vi "SingleJointedArmSim_example.vi"() -> ()   [LabVIEW 2019]
uses:
  <vilib>/Rock Robotics/WPI/ThirdParty/JAS_Junk/TrajLib/DCMOTOR.CTL
  <vilib>/Rock Robotics/WPI/ThirdParty/JAS_Junk/TrajLib/LINEAR_SYSTEM.ctl
  <vilib>/Analysis/Matrix/Datatypes/RealMatrix.ctl
  <vilib>/Rock Robotics/WPI/ThirdParty/JAS_Junk/TrajLib/LINEAR_QUADRATIC_REGULATOR.ctl
  <vilib>/Rock Robotics/WPI/ThirdParty/JAS_Junk/TrajLib/KALMAN_FILTER.ctl
  <vilib>/Rock Robotics/WPI/ThirdParty/JAS_Junk/TrajLib/LINEAR_SYSTEM_LOOP.ctl
  <vilib>/Rock Robotics/WPI/ThirdParty/JAS_Junk/TrajLib/LINEAR_PLANT_INV_FF.ctl
  <vilib>/Rock Robotics/WPI/ThirdParty/JAS_Junk/TrajLib/SINGLE_JOINT_ARM_SIM.ctl
  <vilib>/Rock Robotics/WPI/ThirdParty/JAS_Junk/TrajLib/LINEAR_SYSTEM_SIM.ctl
  <vilib>/numeric/Random Number (Range) DBL.vi
  <vilib>/Rock Robotics/WPI/ThirdParty/JAS_Junk/TrajLib/MatBuilder_Create.vi
  <vilib>/Rock Robotics/WPI/ThirdParty/JAS_Junk/TrajLib/DCMotor_New.vi
  <vilib>/Rock Robotics/WPI/ThirdParty/JAS_Junk/TrajLib/Units_RotationsPerMinuteToRadiansPerSecond.vi
  <vilib>/Rock Robotics/WPI/ThirdParty/JAS_Junk/TrajLib/LinearSystem_New.vi
  <vilib>/Rock Robotics/WPI/ThirdParty/JAS_Junk/TrajLib/MatrixHelper_Zero.vi
  <vilib>/Rock Robotics/WPI/ThirdParty/JAS_Junk/TrajLib/MatBuilder_Fill.vi
  <vilib>/Rock Robotics/WPI/ThirdParty/JAS_Junk/TrajLib/MatrixHelper_CoerceSize.vi
  <vilib>/Rock Robotics/WPI/ThirdParty/JAS_Junk/TrajLib/Trajectory_Library.lvlib
  <vilib>/Analysis/Matrix/NI_Matrix.lvlib
panel:
  in  "Tab Control":T1(tab)
  out "Arm Motor":T2 {"Kt_NMPerAmp" format="%13.5p"; "Kv_RadPerSecPerVolt" format="%13.5p"; "R_Ohms" format="%13.5p"; "FreeSpeed_RadPerSec" format="%13.5p"; "FreeCurrent_Amps" format="%13.5p"; "StallCurrent_Amps" format="%13.5p"; "StallTorque_NM" format="%13.5p"; "nominalVoltage_Volts" format="%13.5p"}
  out "m_Arm":T3
  out "KalmanFilter":T5
  out "Kalman Error":bool
  out "LinearQuadraticRegulator":T6
  out "LQR Error":bool
  out "Linear System Loop":T7
  out "LinSysLoop_Error":bool
  out "Single Joint Arm Simulaation":T9 {"GearBox"."Kt_NMPerAmp" format="%13.5p"; "GearBox"."Kv_RadPerSecPerVolt" format="%13.5p"; "GearBox"."R_Ohms" format="%13.5p"; "GearBox"."FreeSpeed_RadPerSec" format="%13.5p"; "GearBox"."FreeCurrent_Amps" format="%13.5p"; "GearBox"."StallCurrent_Amps" format="%13.5p"; "GearBox"."StallTorque_NM" format="%13.5p"; "GearBox"."nominalVoltage_Volts" format="%13.5p"}
  out "Shooting A":T4
  out "Shooting B":T4
  out "Battery Voltage":dbl format="%20.3f"
  in  "Extra weight":bool
  out "CO Chart":cluster{dbl, "Voltage":dbl}(graph)
  in  "GO UP":bool
  out "Encoer Speed\nRad/Sec":dbl(slide) scale=-1.0..6.0
  out "Height":dbl format="%20.3f"
  out "Cor Err":bool
  out "Kalman Filtered\nHeight":dbl format="%20.3f"
  out "PV Chart":T11(graph)
  out "Predict Err":bool
  out "Motor Volt Dmd (CO)":dbl format="%20.3f"
  out "At Top":bool
  out "At Bottom":bool
  out "Motor Amps":dbl format="%20.3f"
  # "<States,States>"
  # "<States,Inputs>"
  # "<Outputs,States>"
  # "<Outputs,Inputs>"
  # "Steady State Gain  \n<States,Outputs>"
  # "State Estimate <Statess,1>"
  # "<States,States>"
  # "<States,Inputs>"
  # "<Outputs,States>"
  # "<Outputs,Inputs>"
  # "Ref State <States,1>"
  # "Comp and capped \noutput <Inputs,1>"
  # "Controller gain\n<Inputs,States>"
  # "<States,1>"
  # "<FUTURE --- CLAMP TYPE -- For now\nuse Normalize>"
  # "Steady State Gain  \n<States,Outputs>"
  # "State Estimate <Statess,1>"
  # "<States,States>"
  # "<States,Inputs>"
  # "<Outputs,States>"
  # "<Outputs,Inputs>"
  # "<States,1>"
  # "<Inputs,1>"
  # "<States,Inputs>"
  # "<States,States>"
  # "Ref State <States,1>"
  # "Comp and capped \noutput <Inputs,1>"
  # "Controller gain\n<Inputs,States>"
  # "<States, 1>"
  # "<Outputs, 1>"
  # "<Inputs, 1>"
  # "<Outputs, 1>"
  # "<States,States>"
  # "<States,Inputs>"
  # "<Outputs,States>"
  # "<Outputs,Inputs>"
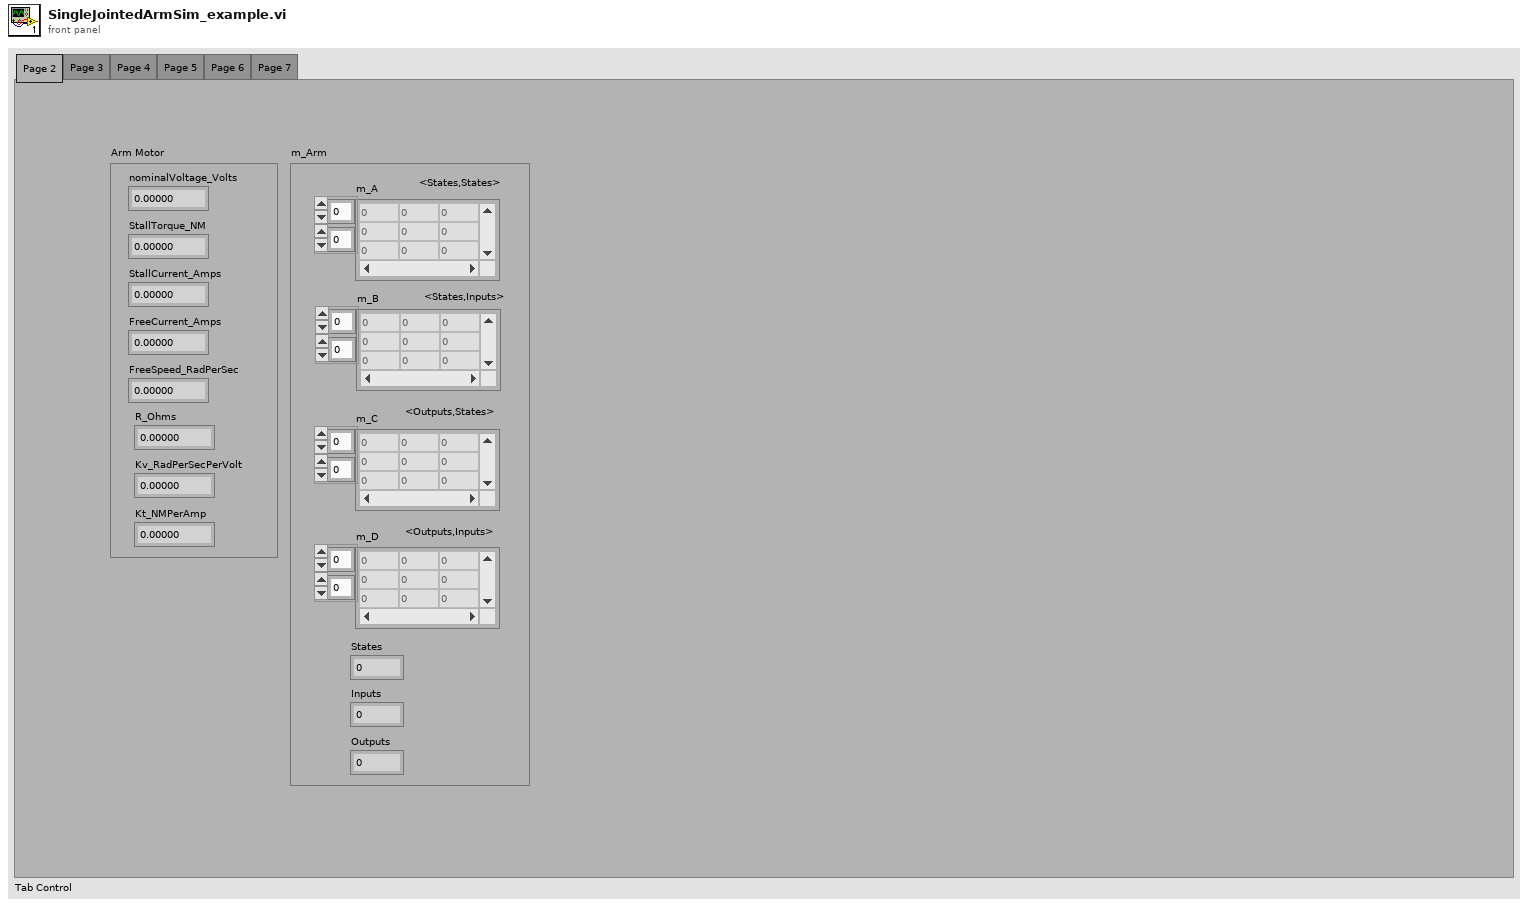
[diagram p1: front panel]
types:
  T1 = enum32{"Page 2", "Page 3", "Page 4", "Page 5", "Page 6", "Page 7"}
  T2 = typedef "Trajectory_Library.lvlib/DCMOTOR.CTL" = cluster{"nominalVoltage_Volts":dbl, "StallTorque_NM":dbl, "StallCurrent_Amps":dbl, "FreeCurrent_Amps":dbl, "FreeSpeed_RadPerSec":dbl, "R_Ohms":dbl, "Kv_RadPerSecPerVolt":dbl, "Kt_NMPerAmp":dbl}
  T3 = typedef "Trajectory_Library.lvlib/LINEAR_SYSTEM.ctl" = cluster{"m_A":T4, "m_B":T4, "m_C":T4, "m_D":T4, "States":i32, "Inputs":i32, "Outputs":i32}
  T4 = typedef "NI_Matrix.lvlib/RealMatrix.ctl" = dbl[][]
  T5 = typedef "Trajectory_Library.lvlib/KALMAN_FILTER.ctl" = cluster{"m_K":T4, "m_xHat":T4, "States":i32, "Outputs":i32, "m_Plant":T3}
  T6 = typedef "Trajectory_Library.lvlib/LINEAR_QUADRATIC_REGULATOR.ctl" = cluster{"m_r":T4, "m_U":T4, "m_K":T4, "States":i32, "Inputs":i32}
  T7 = typedef "Trajectory_Library.lvlib/LINEAR_SYSTEM_LOOP.ctl" = cluster{"Controller":T6, "FeedForward":T8, "Observer":T5, "Next_R":T4, "Clamp Max":T4}
  T8 = typedef "Trajectory_Library.lvlib/LINEAR_PLANT_INV_FF.ctl" = cluster{"m_R":T4, "m_Uff":T4, "m_B":T4, "m_A":T4, "States":i32, "Inputs":i32}
  T9 = typedef "Trajectory_Library.lvlib/SINGLE_JOINT_ARM_SIM.ctl" = cluster{"Arm_LinearSystem":T10, "GearBox":T2, "Gearing":dbl, "R_ArmLength_M":dbl, "MinAngle_M":dbl, "MaxAngle_M":dbl, "ArmMass_Kg":dbl, "SimulateGravity":bool}
  T10 = typedef "Trajectory_Library.lvlib/LINEAR_SYSTEM_SIM.ctl" = cluster{"m_Plant":T3, "m_X":T4, "m_Y":T4, "m_U":T4, "MeasureStdDev":T4}
  T11 = cluster{"upper limit":dbl, "Real Matrix Element":dbl, "Real Matrix Element":dbl}
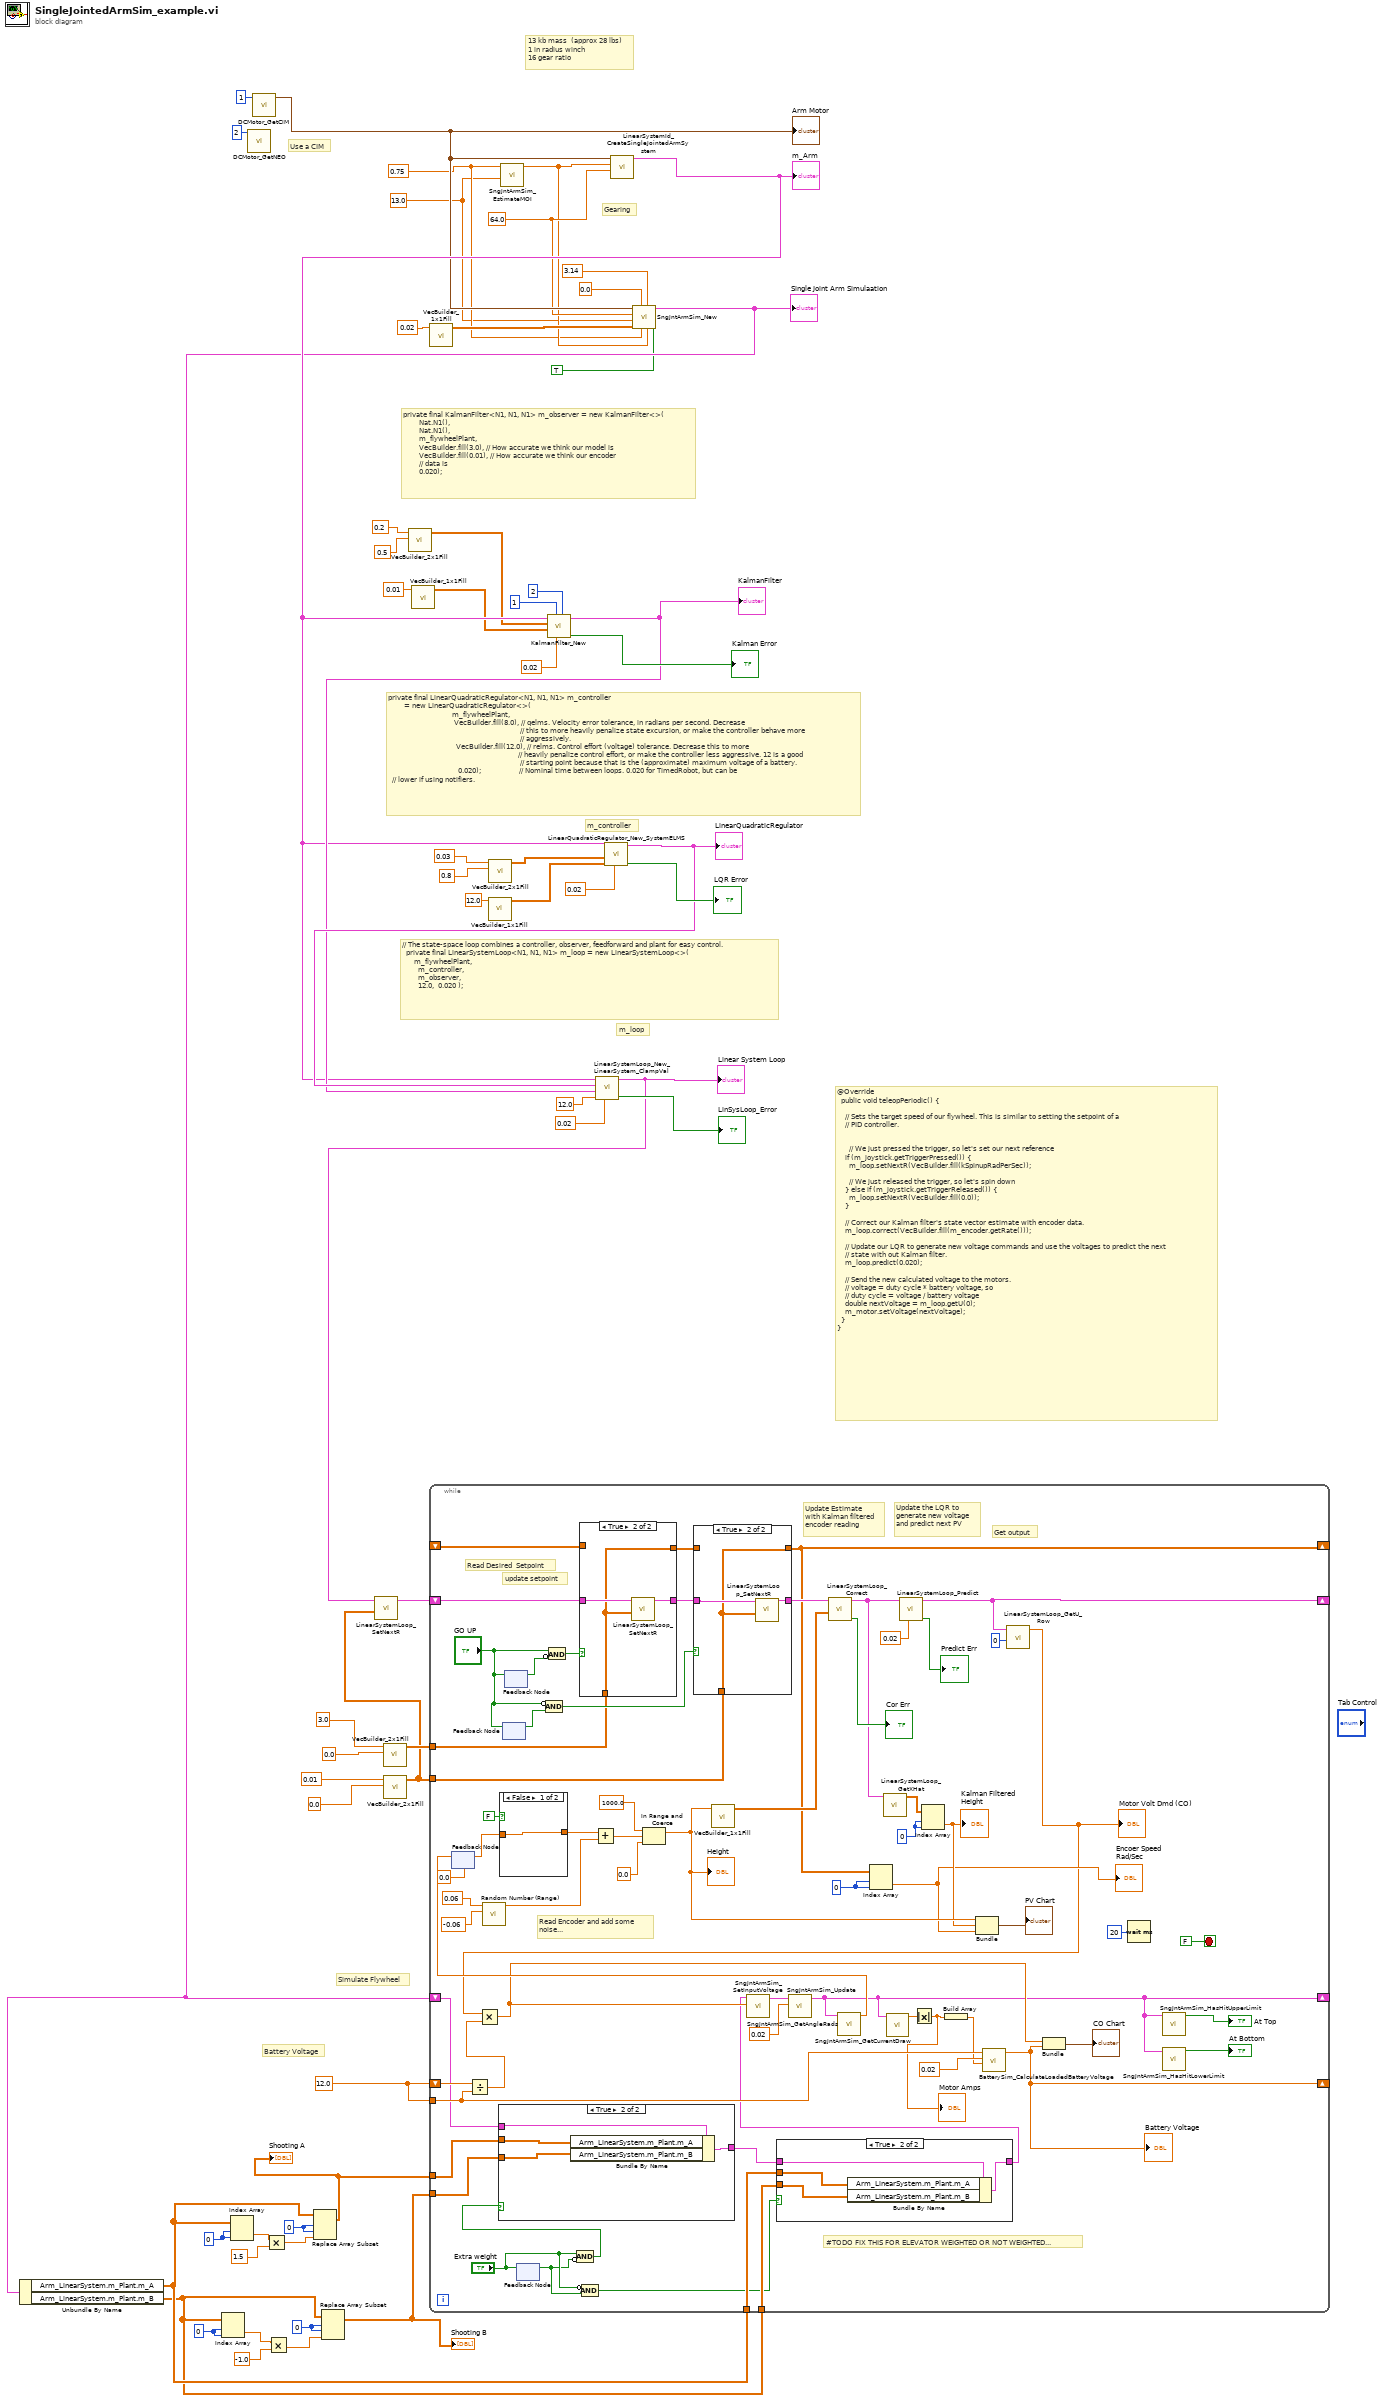
[diagram p0: block diagram]
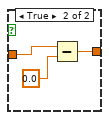
[diagram p4: hidden frame]
diagram:
  w3 = 0.75 ("ArmLength_M")
  w23 = 0 ("index (row)")
  w24 = 0 ("index (row)")
  w25 = 0 ("index (row)")
  w26 = 0 ("index (row)")
  w6 = 64.0 ("G")
  w2 = 13.0 ("massKg")
  w50 = 12.0
  # "Simulate Flywheel"
  # "m_loop"
  # "m_controller"
  # "13 kb mass  (approx 28 lbs)\n1 in radius winch\n16 gear ratio"
  # "Gearing"
  # "Use a CIM"
  # "Battery Voltage"
  # "@Override\n  public void teleopPeriodic() {\n\n    // Sets the target speed of our flywheel. This is similar to setting the setpoint of a\n    // PID controller.\n\n\n      // We just pressed the trigger, so let's set our next reference\n    if (m_joystick.getTriggerPressed()) {\n      m_loop.setNextR(VecBuilder.fill(kSpinupRadPerSec));\n\n      // We just released the trigger, so let's spin down\n    } else if (m_joystick.getTriggerReleased()) {\n      m_loop.setNextR(VecBuilder.fill(0.0));\n    }\n\n    // Correct our Kalman filter's state vector estimate with encoder data.\n    m_loop.correct(VecBuilder.fill(m_encoder.getRate()));\n\n    // Update our LQR to generate new voltage commands and use the voltages to predict the next\n    // state with out Kalman filter.\n    m_loop.predict(0.020);\n\n    // Send the new calculated voltage to the motors.\n    // voltage = duty cycle * battery voltage, so\n    // duty cycle = voltage / battery voltage\n    double nextVoltage = m_loop.getU(0);\n    m_motor.setVoltage(nextVoltage);\n  }\n}"
  # "// The state-space loop combines a controller, observer, feedforward and plant for easy control.\n  private final LinearSystemLoop<N1, N1, N1> m_loop = new LinearSystemLoop<>(\n      m_flywheelPlant,\n        m_controller,\n        m_observer,\n        12.0,  0.020 );"
  # "private final LinearQuadraticRegulator<N1, N1, N1> m_controller\n        = new LinearQuadraticRegulator<>(\n                                m_flywheelPlant,\n                                 VecBuilder.fill(8.0), // qelms. Velocity error tolerance, in radians per second. Decrease\n                                                                  // this to more heavily penalize state excursion, or make the controller behave more\n                                                                  // aggressively.\n                                  VecBuilder.fill(12.0), // relms. Control effort (voltage) tolerance. Decrease this to more\n                                                                 // heavily penalize control effort, or make the controller less aggressive. 12 is a good\n                                                                  // starting point because that is the (approximate) maximum voltage of a battery.\n                                   0.020);                   // Nominal time between loops. 0.020 for TimedRobot, but can be\n  // lower if using notifiers."
  # "private final KalmanFilter<N1, N1, N1> m_observer = new KalmanFilter<>(\n        Nat.N1(), \n        Nat.N1(),\n        m_flywheelPlant,\n        VecBuilder.fill(3.0), // How accurate we think our model is\n        VecBuilder.fill(0.01), // How accurate we think our encoder\n        // data is\n        0.020);"
  n1 = call <vilib>:"DCMotor_GetNEO.vi"("Num Motors"=2) -> ()  [unwired: 10 in, 1 out]
  n2 = call <vilib>:"DCMotor_GetCIM.vi"("Num Motors"=1) -> ("DCMOTOR"=w9:T2)  [unwired: 10 in]
  "Arm Motor" <- w9
  n3 = call <vilib>:"VecBuilder_2x1Fill.vi"("R1"=0.0, "R0"=3.0 ("RotationsPerMinute")) -> ("output matrix"=w16:T4)  [unwired: 9 in]
  n4 = call <vilib>:"VecBuilder_2x1Fill.vi"("R1"=0.0, "R0"=0.01 ("R0_C0")) -> ("output matrix"=w11:T4)  [unwired: 9 in]
  n5 = call <vilib>:"VecBuilder_2x1Fill.vi"("R1"=0.5, "R0"=0.2 ("R0_C0")) -> ("output matrix"=w37:T4)  [unwired: 9 in]
  n6 = call <vilib>:"VecBuilder_1x1Fill.vi"("R0_C0"=0.01) -> ("output matrix"=w36:T4)  [unwired: 10 in]
  n7 = call <vilib>:"VecBuilder_1x1Fill.vi"("R0_C0"=0.02) -> ("output matrix"=w5:T4)  [unwired: 10 in]
  n8 = call <vilib>:"VecBuilder_1x1Fill.vi"("R0_C0"=12.0) -> ("output matrix"=w30:T4)  [unwired: 10 in]
  n9 = call <vilib>:"VecBuilder_2x1Fill.vi"("R1"=0.8 ("R0_C0"), "R0"=0.03 ("R0_C0")) -> ("output matrix"=w32:T4)  [unwired: 9 in]
  n10 = call <vilib>:"SngJntArmSim_EstimateMOI.vi"("ArmMass_Kg"=w2, "ArmLength_M"=w3) -> ("MOI"=w4:dbl)  [unwired: 9 in]
  n11 = call <vilib>:"LinearSystemId_CreateSingleJointedArmSystem.vi"("G"=w6, "jKgSquaredMeters"=w4, "DCMOTOR"=w9) -> ("Linearsystem"=w44:T3)  [unwired: 8 in]
  "m_Arm" <- w44
  n12 = call <vilib>:"KalmanFilter_New.vi"("States"=2, "dt_Seconds"=0.02, "Outputs"=1, "MeasurementStdDevs"=w36, "StateStdDevs"=w37, "Plant"=w44) -> ("Error"=→"Kalman Error":bool, "KalmanFilter"=w54:T5)  [unwired: 4 in]
  "KalmanFilter" <- w54
  n13 = call <vilib>:"LinearQuadraticRegulator_New_SystemELMS.vi"("dt_Seconds"=0.02, "Relms"=w30, "Qelms"=w32, "LINEARSYSTEM"=w44) -> ("Error"=→"LQR Error":bool, "LinearQuadraticRegulator"=w55:T6)  [unwired: 6 in]
  "LinearQuadraticRegulator" <- w55
  n14 = call <vilib>:"LinearSystemLoop_New_LinearSystem_ClampVal.vi"("dT_Seconds"=0.02, "Max_Voltage"=12.0, "Observer"=w54, "Controller"=w55, "Plant"=w44) -> ("Error"=→"LinSysLoop_Error":bool, "Linear System Loop"=w12:T7)  [unwired: 5 in]
  "Linear System Loop" <- w12
  n15 = call <vilib>:"LinearSystemLoop_SetNextR.vi"("R"=w11, "input inear System Loop"=w12) -> ("out Linear System Loop"=w13:T7)  [unwired: 9 in]
  n16 = call <vilib>:"SngJntArmSim_New.vi"("SimulateGravity"=TRUE, "jKgMetersSquared"=w4, "MaxAngle_Rad"=3.14 ("MaxHeight_Meters"), "ArmLength_Meters"=w3, "MinAngle_Rad"=0.0 ("MinHeight_Meters"), "MeasurementStdDev"=w5, "ArmMass_Kg"=w2, "Gearing"=w6, "GearBox"=w9) -> ("SingleJointArmSim"=w10:T9)  [unwired: 2 in]
  "Single Joint Arm Simulaation" <- w10
  n17 = Unbundle By Name(w10) -> ("Arm_LinearSystem.m_Plant.m_A"=w48:T4, "Arm_LinearSystem.m_Plant.m_B"=w47:T4)
  n18 = Index Array(array=w47, index (row)=w26, index (col)=w26) -> (element=w18:dbl)
  n19 = Index Array(array=w48, index (row)=w25, index (col)=w25) -> (element=w22:dbl)
  n20 = Multiply(x=w22, y=1.5) -> (x*y=w20:dbl)
  n21 = Multiply(x=w18, y=-1.0) -> (x*y=w17:dbl)
  n22 = Replace Array Subset(array=w48, new element=w20, index (row)=w23, index (col)=w23) -> (w46:T4)
  "Shooting A" <- w46
  n23 = Replace Array Subset(array=w47, new element=w17, index (row)=w24, index (col)=w24) -> (w45:T4)
  "Shooting B" <- w45
  n24 = while {
    shift-right: [w68] -> _
    shift-left: w13 -> [w118]
    tunnel: w16 -> [w116]
    tunnel: w11 -> [w115]
    shift-right: [w59] -> _
    shift-left: w10 -> [w76]
    shift-right: [w90] -> _
    shift-left: _ -> [w91]
    shift-right: [w78] -> _
    shift-left: w50 -> [w85]
    tunnel: w50 -> [w82]
    tunnel: w48 -> [w72]
    tunnel: w47 -> [w71]
    tunnel: w46 -> [w70]
    tunnel: w45 -> [w69]
    stop <- FALSE stop-if-true
    w89 = 0 ("index (row)")
    w105 = 0 ("index (row)")
    # "#TODO FIX THIS FOR ELEVATOR WEIGHTED OR NOT WEIGHTED..."
    # "Get output"
    # "Update the LQR to \ngenerate new voltage\nand predict next PV"
    # "update setpoint"
    # "Read Desired  Setpoint"
    # "Update Estimate\nwith Kalman filtered\nencoder reading"
    # "Read Encoder and add some \nnoise..."
    n25 = feedback #1(0.0 ("Velocity_RadPerSec")) -> (w87:dbl)
    n26 = Divide(x=w85, y=w82) -> (x/y=w83:dbl)
    n27 = call-poly <vilib>:"Random Number (Range).vi"("lower bound (0)"=-0.06, "upper bound (100)"=0.06) -> ("number"=w112:dbl)  [unwired: 9 in]
    n28 = case shown="False" FALSE {
      tunnel: w87 -> [w136 w139]
      tunnel: [w136 w138] -> w86
      frame False {
      }
      frame True {
        n29 = Subtract(x=w139, y=0.0) -> (x-y=w138:dbl)
      }
    }
    n30 = feedback #2() -> (w122:bool)  [unwired: 1 in]
    n31 = feedback-in #2("GO UP") -> ()
    n32 = feedback-in #3("GO UP") -> ()
    n33 = feedback #3() -> (w123:bool)  [unwired: 1 in]
    n34 = feedback-in #4("Extra weight") -> ()
    n35 = feedback #4() -> (w64:bool)  [unwired: 1 in]
    n36 = Compound Arithmetic op=AND(invert "GO UP", w122) -> (w119:bool)
    n37 = Compound Arithmetic op=AND("GO UP", invert w123) -> (w120:bool)
    n38 = Compound Arithmetic op=AND("Extra weight", invert w64) -> (w73:bool)
    n39 = case shown="True" w73 {
      tunnel: w76 -> [w131 w135]
      tunnel: [w131 w132] -> w75
      tunnel: w70 -> [_ w134]
      tunnel: w69 -> [_ w133]
      frame False {
      }
      frame True {
        n40 = Bundle By Name(cluster=w135, "Arm_LinearSystem.m_Plant.m_A"=w134, "Arm_LinearSystem.m_Plant.m_B"=w133) -> (w132:T9)
      }
    }
    n41 = case shown="True" w120 {
      tunnel: w118 -> [w146 w148]
      tunnel: [w146 w149] -> w117
      tunnel: w116 -> [_ w147]
      tunnel: [w145 w147] -> w92
      tunnel: w91 -> [w145 _]
      frame False {
      }
      frame True {
        n42 = call <vilib>:"LinearSystemLoop_SetNextR.vi"("R"=w147, "input inear System Loop"=w148) -> ("out Linear System Loop"=w149:T7)  [unwired: 9 in]
      }
    }
    n43 = Compound Arithmetic op=AND(invert "Extra weight", w64) -> (w63:bool)
    n44 = Add(x=w86, y=w112) -> (x+y=w110:dbl)
    n45 = In Range and Coerce(upper limit=1000.0, x=w110, lower limit=0.0) -> (coerced(x)=w103:dbl)  [unwired: 1 out]
    "Height" <- w103
    n46 = case shown="True" w119 {
      tunnel: w117 -> [w141 w143]
      tunnel: [w141 w144] -> w108
      tunnel: w115 -> [_ w142]
      tunnel: w92 -> [w140 _]
      tunnel: [w140 w142] -> w90
      frame False {
      }
      frame True {
        n47 = call <vilib>:"LinearSystemLoop_SetNextR.vi"("R"=w142, "input inear System Loop"=w143) -> ("out Linear System Loop"=w144:T7)  [unwired: 9 in]
      }
    }
    n48 = call <vilib>:"VecBuilder_1x1Fill.vi"("R0_C0"=w103) -> ("output matrix"=w107:T4)  [unwired: 10 in]
    n49 = case shown="True" w63 {
      tunnel: w75 -> [w126 w130]
      tunnel: [w126 w129] -> w60
      tunnel: w72 -> [_ w128]
      tunnel: w71 -> [_ w127]
      frame False {
      }
      frame True {
        n50 = Bundle By Name(cluster=w130, "Arm_LinearSystem.m_Plant.m_A"=w128, "Arm_LinearSystem.m_Plant.m_B"=w127) -> (w129:T9)
      }
    }
    n51 = call <vilib>:"LinearSystemLoop_Correct.vi"("Y"=w107, "input inear System Loop"=w108) -> ("Error"=→"Cor Err":bool, "out Linear System Loop"=w100:T7)  [unwired: 8 in]
    n52 = Index Array(array=w90, index (row)=w89, index (col)=w89) -> (element=w88:dbl)
    "Encoer Speed\nRad/Sec" <- w88
    n53 = call <vilib>:"LinearSystemLoop_GetXHat.vi"("input inear System Loop"=w100) -> ("XHat"=w104:T4)  [unwired: 10 in]
    n54 = call <vilib>:"LinearSystemLoop_Predict.vi"("dT_Seconds"=0.02, "input inear System Loop"=w100) -> ("Error"=→"Predict Err":bool, "out Linear System Loop"=w68:T7)  [unwired: 8 in]
    n55 = Index Array(array=w104, index (row)=w105, index (col)=w105) -> (element=w102:dbl)
    "Kalman Filtered\nHeight" <- w102
    n56 = Bundle("upper limit"=w103, "Real Matrix Element"=w102, "Real Matrix Element"=w88) -> (→"PV Chart":T11)  [unwired: 1 in]
    n57 = call <vilib>:"LinearSystemLoop_GetU_Row.vi"("Row"=0, "input inear System Loop"=w68) -> ("U"=w84:dbl)  [unwired: 9 in]
    "Motor Volt Dmd (CO)" <- w84
    n58 = Multiply(x=w84, y=w83) -> (x*y=w77:dbl)
    n59 = call <vilib>:"SngJntArmSim_SetInputVoltage.vi"("Input_Voltage"=w77, "in SingleJointArmSim"=w60) -> ("out SingleJointArmSim"=w96:T9)  [unwired: 9 in]
    n60 = call <vilib>:"SngJntArmSim_Update.vi"("dT_Seconds"=0.02, "in SingleJointArmSim"=w96) -> ("out SingleJointArmSim"=w59:T9)  [unwired: 9 in]
    n61 = call <vilib>:"SngJntArmSim_GetAngleRads.vi"("SingleJointArmSim"=w59) -> ("ArmAngle_Rad"=w94:dbl)  [unwired: 10 in]
    n62 = feedback-in #1(w94) -> ()
    n63 = call <vilib>:"SngJntArmSim_GetCurrentDraw.vi"("SingleJointArmSim"=w59) -> ("Current_Amps"=w62:dbl)  [unwired: 10 in]
    n64 = Absolute Value(x=w62) -> (abs(x)=w61:dbl)
    "Motor Amps" <- w61
    n65 = Build Array(w61) -> (w80:dbl[])
    n66 = call <vilib>:"BatterySim_CalculateLoadedBatteryVoltage.vi"("Currents"=w80, "Resistance_Ohms"=0.02, "NominalVoltage"=w82) -> ("Voltage"=w78:dbl)  [unwired: 8 in]
    "Battery Voltage" <- w78
    n67 = Bundle(w77, "Voltage"=w78) -> (→"CO Chart":cluster{dbl, "Voltage":dbl})  [unwired: 1 in]
    n68 = Wait (ms)(milliseconds to wait=u32 20) -> ()  [unwired: 1 out]
    n69 = call <vilib>:"SngJntArmSim_HasHitUpperLimit.vi"("SingleJointArmSim"=w59) -> ("At HIgh LImit"=→"At Top":bool)  [unwired: 10 in]
    n70 = call <vilib>:"SngJntArmSim_HasHitLowerLimit.vi"("SingleJointArmSim"=w59) -> ("AtLowLimit"=→"At Bottom":bool)  [unwired: 10 in]
  }
